vi "Get Key Value (Control Value).vi"(5 "Key name":string, 6 "Control reference":refnum<vi>, 7 "Section name":string, 8 "error in (no error)":errorcluster, 9 "Use LV Default? [F]":bool, 10 "Value signaling? [F]":bool, 11 "Carya Config in":refnum<class "Carya Config.lvclass">) -> (0 "error out":errorcluster, 1 "Found?":bool, 2 "Value":variant, 3 "Carya Config out":refnum<class "Carya Config.lvclass">)   [LabVIEW 2013, in "Carya Config.lvclass"]
doc: "Copyright 2018, Carya Automatisering, Wiebe Walstra."
uses:
  Carya Config.lvclass
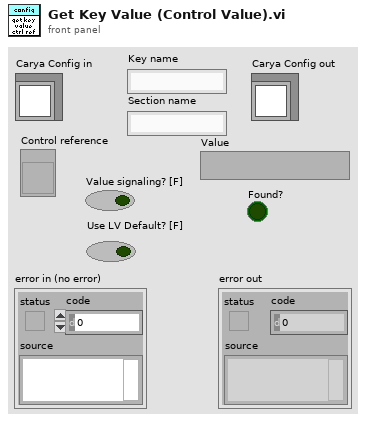
[diagram p1: front panel]
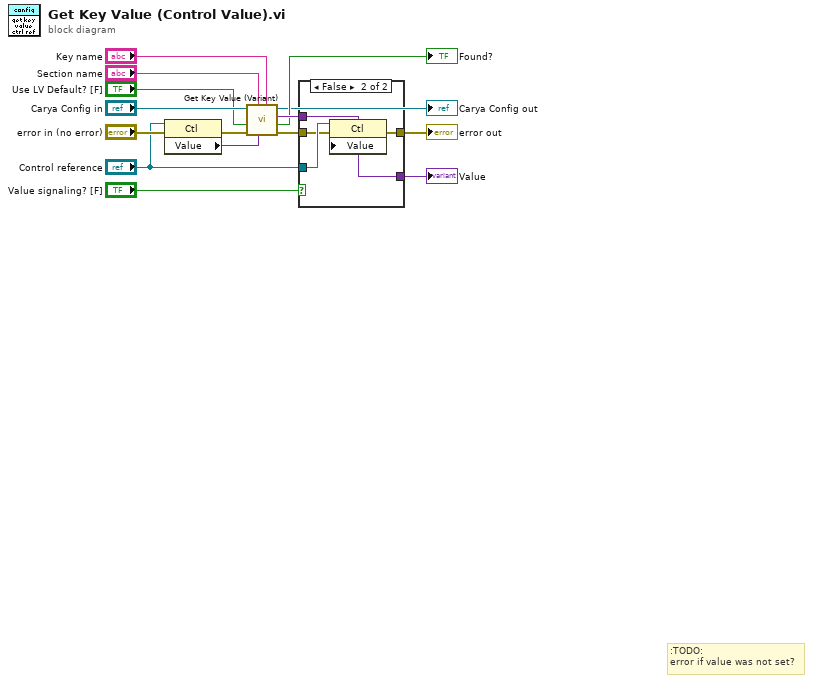
[diagram p0: block diagram]
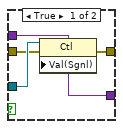
[diagram p2: hidden frame]
diagram:
  # ":TODO:\nerror if value was not set?"
  n1 = property class="Ctl"(reference="Control reference", error in="error in (no error)") -> (error out=w7:errorcluster, "Value"=w5:variant)  [unwired: 1 out]
  n2 = call "Get Key Value (Variant).vi"("Key name"="Key name", "Default value"=w5, "Section name"="Section name", "error in (no error)"=w7, "Use LV Default? [F]"="Use LV Default? [F]", "Carya Config in"="Carya Config in") -> ("error out"=w14:errorcluster, "Found?"=→"Found?":bool, "Value"=w9:variant, "Carya Config out"=→"Carya Config out":refnum<class "Carya Config.lvclass">)  [unwired: 2 in]
  n3 = case shown="False" "Value signaling? [F]" {
    tunnel: w14 -> [w18 w22]
    tunnel: [w17 w21] -> w10
    tunnel: w9 -> [w16 w20]
    tunnel: "Control reference" -> [w19 w23]
    tunnel: [w16 w20] -> w3
    frame True {
      n4 = property class="Ctl"(reference=w19, error in=w18, "Val(Sgnl)"=w16) -> (error out=w17:errorcluster)  [unwired: 1 out]
    }
    frame False {
      n5 = property class="Ctl"(reference=w23, error in=w22, "Value"=w20) -> (error out=w21:errorcluster)  [unwired: 1 out]
    }
  }
  "error out" <- w10
  "Value" <- w3
